vi "Log Info(by Ref).vi"(10 "error in (no error)":errorcluster, 11 "Message":string) -> (2 "error out":errorcluster)   [LabVIEW 2017, in "Error Log.lvlib" / "Logger.lvclass"]
doc: "Logs an event with level <b>Info</b> to the referenced Logger."
uses:
  Logger.lvclass
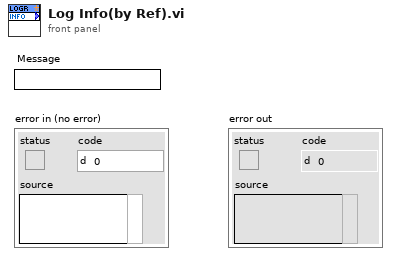
[diagram p1: front panel]
types:
  T1 = enum16{"DEBUG", "INFO", "WARNING", "ERROR", "CRITICAL"}
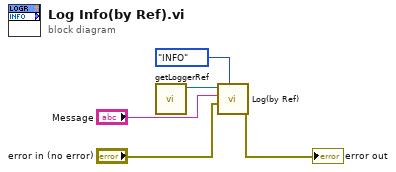
[diagram p0: block diagram]
diagram:
  n1 = call "getLoggerRef.vi"() -> ("Logger Ref"=w3:refnum<data-value>)  [unwired: 10 in, 1 out]
  n2 = call "Log(by Ref).vi"("Level"=T1."INFO", "error"="error in (no error)", "Message"="Message", "Logger Ref in"=w3) -> ("error out"=→"error out":errorcluster)  [unwired: 6 in, 1 out]
